vi "Wait Time.vi"(0 "Delay Time (s)":dbl=0.5, 11 "error in":errorcluster, 13 "Set Time":bool) -> (15 "error out":errorcluster)   [LabVIEW 2017, in "I28Drivers.lvlib"]
uses:
  I28Drivers.lvlib
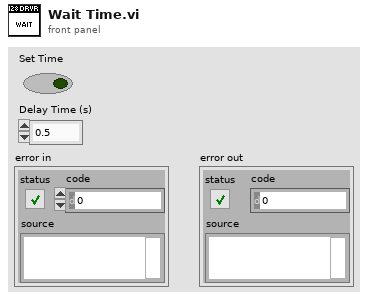
[diagram p1: front panel]
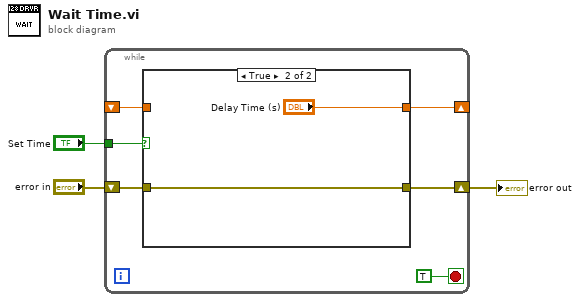
[diagram p0: block diagram]
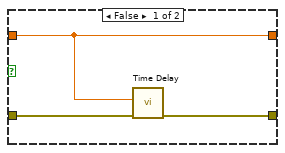
[diagram p2: hidden frame]
diagram:
  n1 = while {
    shift-right: [w8] -> w2
    shift-left: "error in" -> [w9]
    tunnel: "Set Time" -> [w6]
    shift-right: [w5] -> _
    shift-left: _ -> [w4]
    stop <- TRUE stop-if-true
    n2 = case shown="True" w6 {
      tunnel: w9 -> [w12 w13]
      tunnel: [w11 w13] -> w8
      tunnel: w4 -> [w10 _]
      tunnel: [w10 "Delay Time (s)"] -> w5
      frame False {
        n3 = call "Time Delay"("error in (no error)"=w12, "Delay Time (s)"=w10) -> ("error out"=w11:errorcluster)  [unwired: 9 in]
      }
      frame True {
      }
    }
  }
  "error out" <- w2
